vi "Read 02-05.vi"() -> (3 "02-05-9205":dbl[](array[numeric]))   [LabVIEW 2018]
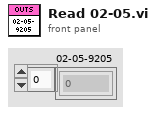
[diagram p1: front panel]
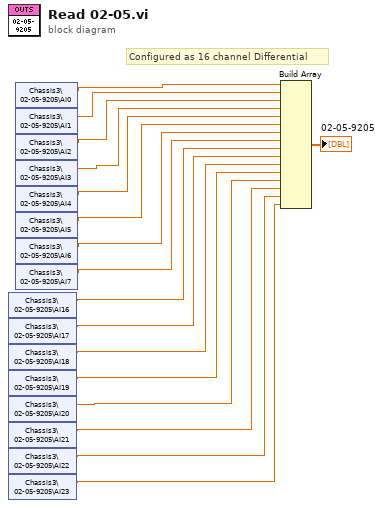
[diagram p0: block diagram]
diagram:
  # "Configured as 16 channel Differential"
  n1 = shared-variable "Chassis3\\02-05-9205\\AI16"() -> (w8:dbl)  [unwired: 1 in, 1 out]
  n2 = shared-variable "Chassis3\\02-05-9205\\AI17"() -> (w7:dbl)  [unwired: 1 in, 1 out]
  n3 = shared-variable "Chassis3\\02-05-9205\\AI18"() -> (w6:dbl)  [unwired: 1 in, 1 out]
  n4 = shared-variable "Chassis3\\02-05-9205\\AI19"() -> (w5:dbl)  [unwired: 1 in, 1 out]
  n5 = shared-variable "Chassis3\\02-05-9205\\AI20"() -> (w4:dbl)  [unwired: 1 in, 1 out]
  n6 = shared-variable "Chassis3\\02-05-9205\\AI21"() -> (w3:dbl)  [unwired: 1 in, 1 out]
  n7 = shared-variable "Chassis3\\02-05-9205\\AI22"() -> (w2:dbl)  [unwired: 1 in, 1 out]
  n8 = shared-variable "Chassis3\\02-05-9205\\AI23"() -> (w1:dbl)  [unwired: 1 in, 1 out]
  n9 = shared-variable "Chassis3\\02-05-9205\\AI0"() -> (w16:dbl)  [unwired: 1 in, 1 out]
  n10 = shared-variable "Chassis3\\02-05-9205\\AI1"() -> (w15:dbl)  [unwired: 1 in, 1 out]
  n11 = shared-variable "Chassis3\\02-05-9205\\AI2"() -> (w14:dbl)  [unwired: 1 in, 1 out]
  n12 = shared-variable "Chassis3\\02-05-9205\\AI3"() -> (w13:dbl)  [unwired: 1 in, 1 out]
  n13 = shared-variable "Chassis3\\02-05-9205\\AI4"() -> (w12:dbl)  [unwired: 1 in, 1 out]
  n14 = shared-variable "Chassis3\\02-05-9205\\AI5"() -> (w11:dbl)  [unwired: 1 in, 1 out]
  n15 = shared-variable "Chassis3\\02-05-9205\\AI6"() -> (w10:dbl)  [unwired: 1 in, 1 out]
  n16 = shared-variable "Chassis3\\02-05-9205\\AI7"() -> (w9:dbl)  [unwired: 1 in, 1 out]
  n17 = Build Array(w16, w15, w14, w13, w12, w11, w10, w9, w8, w7, w6, w5, w4, w3, w2, w1) -> (→"02-05-9205":dbl[])
